vi "get data definition.vi"(10 "channel classification":T1, 11 "fixed channel runtime in":refnum<class "Watchdog runtime.lvclass">) -> (1 "valid?":bool, 2 "index cluster":variant, 3 "fixed channel runtime out":refnum<class "Watchdog runtime.lvclass">)   [LabVIEW 2013, in "Watchdog runtime.lvclass"]
uses:
  Watchdog runtime.lvclass
  <vilib>/NI/Tag Bus Module Framework/channel/channel classification.ctl
  <vilib>/NI/DCAF/Tag Editor Core/control module/runtime/control module runtime.lvclass
  <vilib>/NI/Tag Bus Module Framework/channel/TBM channel.lvclass
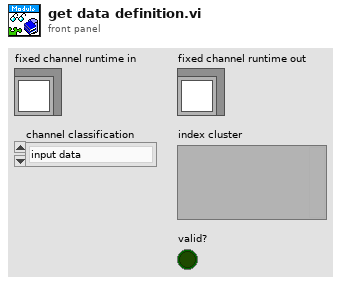
[diagram p1: front panel]
types:
  T1 = typedef "TBM channel.lvclass/channel classification.ctl" = enum16{"input data", "output data", "processing parameter", "processing result"}
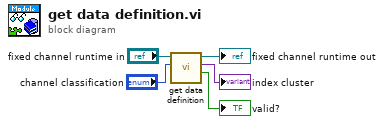
[diagram p0: block diagram]
diagram:
  n1 = call-parent "get data definition.vi"("channel classification"="channel classification", "fixed channel runtime in"="fixed channel runtime in") -> ("valid?"=→"valid?":bool, "index cluster"=→"index cluster":variant, "fixed channel runtime out"=→"fixed channel runtime out":refnum<class "Watchdog runtime.lvclass">)  [unwired: 7 in]
